vi "Linear Length 1 1721 1853.vi"(6 "Calibration Image":T2, 7 "error in":errorcluster, 8 "ROI 2 Parameters":T9={"ROI 2 Descriptor"={"Global Rectangle"=[], "Contours"=[]}, " ROI 2 Step Size"=10, "ROI 2 Scan Direction"=0, "ROI 2 Process"=enum."Get First + Last Edge", "ROI 2 Edge Options"={"Edge Polarity"=0, "Kernel Size"=3, "Width"=3, "Minimum Edge Strength"=40.0, "Interpolation Type"=enum."Zero Order", "Data Processing Method"=enum."Average"}, "ROI 2 Overlay"=TRUE, "ROI 2 Rake Line Overlay"=TRUE, "ROI 2 Edge/Point Overlay"=TRUE} {"ROI 2 Descriptor"."Contours"."Type" items=["No Selection", "Point", "Line", "Rectangle", "Oval", "Polygon", "Freehand Region", "Annulus", "Unused2", "Unused3", "Broken Line", "Freehand Line", "Rotated Rectangle"]; "ROI 2 Scan Direction" items=["Left To Right", "Right To Left", "Top To Bottom", "Bottom To Top"]; "ROI 2 Edge Options"."Edge Polarity" items=["All Edges", "Rising Edges", "Falling Edges"]; "ROI 2 Edge Options"."Minimum Edge Strength" format="%.2f"; "ROI 2 Edge Options"."Width" step=2; "ROI 2 Edge Options"."Kernel Size" step=2}, 9 "ROI 1 Parameters":T7={"ROI 1 Descriptor"={"Global Rectangle"=[], "Contours"=[]}, "ROI 1 Line Options"={"Number of Lines"=1, "Type"=enum."Best Edge Rake", "Min. Score"=10.0, "Max. Score"=1000.0, "Orientation"=0.0, "Angle Range"=10.0, "Angle Tolerance"=1.0, "Step Size"=5, "Min. SNR (db)"=0.0, "Min. Points (%)"=25.0, "Hough Iterations"=5}, "ROI 1 Edge Options"={"Edge Polarity"=2, "Kernel Size"=3, "Width"=3, "Minimum Edge Strength"=25.0, "Interpolation Type"=enum."Zero Order", "Data Processing Method"=enum."Average"}, "ROI 1 Search Direction"=1, "ROI 1 Overlay"=TRUE, "ROI 1 Rake Line Overlay"=TRUE, "ROI 1 Edge/Point Overlay"=TRUE} {"ROI 1 Descriptor"."Contours"."Type" items=["No Selection", "Point", "Line", "Rectangle", "Oval", "Polygon", "Free", "Annulus", "Unused2", "Unused3", "Broken Line", "Free Hand Line", "Rotated Rectangle"]; "ROI 1 Line Options"."Min. Points (%)" min=0.0 max=100.0; "ROI 1 Line Options"."Min. SNR (db)" min=0.0; "ROI 1 Line Options"."Max. Score" min=0.0 max=1024.0; "ROI 1 Line Options"."Min. Score" min=0.0 max=1024.0 step=1.0; "ROI 1 Edge Options"."Edge Polarity" items=["All Edges", "Rising Edges", "Falling Edges"]; "ROI 1 Edge Options"."Minimum Edge Strength" format="%.2f"; "ROI 1 Edge Options"."Width" step=2; "ROI 1 Edge Options"."Kernel Size" step=2; "ROI 1 Search Direction" items=["Left to Right", "Right to Left", "Top to Bottom", "Bottom to Top"]}, 10 "Input Image":T2) -> (0 "error  out":errorcluster, 1 "Overlay Arrow Lines":T1, 2 "L Outputs":T10, 3 "Refnum out":T2(plugin-control))   [LabVIEW 2019, in "Algorithm.lvclass"]
doc: "Using L advance Line ROI and L advance Search Direction find straight line.\nFind 2 Left Corner Edge points using Rake3 with right inputs. Again find left corner point between these points.\nCalculate perpendicular distance from this point to the line."
uses:
  FrameworkOverrides/Algorithm.lvclass
  <vilib>/vision/NI_Vision_Development_Module.lvlib
  <vilib>/vision/Measure.llb/Edge Polarity.ctl
  <vilib>/vision/Measure.llb/Edge Options.ctl
  <vilib>/vision/Measure.llb/Straight Edge Process.ctl
  <vilib>/vision/Measure.llb/Straight Edge Options.ctl
  <vilib>/vision/Image Controls.llb/IMAQ Image.ctl
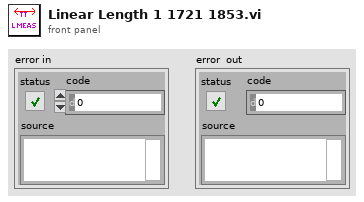
[diagram p1: front panel]
types:
  T1 = cluster{"First Overlay Line ":cluster{"Start Point":cluster{"X":sgl, "Y":sgl}, "Start Point":cluster{"X":sgl, "Y":sgl}}, "Second Overlay Line ":cluster{"Start Point":cluster{"X":sgl, "Y":sgl}, "Start Point":cluster{"X":sgl, "Y":sgl}}}
  T2 = typedef "IMAQ Image.ctl" = refnum<image>
  T3 = typedef "Straight Edge Options.ctl" = cluster{"Number of Lines":i32, "Type":T4, "Min. Score":dbl, "Max. Score":dbl, "Orientation":dbl, "Angle Range":dbl, "Angle Tolerance":dbl, "Step Size":u32, "Min. SNR (db)":dbl, "Min. Points (%)":dbl, "Hough Iterations":i32}
  T4 = typedef "Straight Edge Process.ctl" = enum32{"First Edge Rake", "Best Edge Rake", "Hough Edge Rake", "First Edge Projection", "Best Edge Projection"}
  T5 = typedef "Edge Options.ctl" = cluster{"Edge Polarity":T6, "Kernel Size":u32, "Width":u32, "Minimum Edge Strength":sgl, "Interpolation Type":enum32{"Zero Order", "Bilinear", "Quadratic", "Cubic", "Bilinear Fixed"}, "Data Processing Method":enum32{"Average", "Median"}}
  T6 = typedef "Edge Polarity.ctl" = u32
  T7 = cluster{"ROI 1 Descriptor":cluster{"Global Rectangle":i32[], "Contours":cluster{"ID":enum32{"External", "Internal"}, "Type":u32, "Coordinates":i32[]}[]}, "ROI 1 Line Options":T3, "ROI 1 Edge Options":T5, "ROI 1 Search Direction":u32, "ROI 1 Overlay":bool, "ROI 1 Rake Line Overlay":bool, "ROI 1 Edge/Point Overlay":bool}
  T8 = typedef "ROI Descriptor" = cluster{"Global Rectangle":i32[], "Contours":cluster{"ID":enum32{"External", "Internal"}, "Type":u32, "Coordinates":i32[]}[]}
  T9 = cluster{"ROI 2 Descriptor":T8, " ROI 2 Step Size":u32, "ROI 2 Scan Direction":u16, "ROI 2 Process":enum16{"Get First Edge", "Get First + Last Edge", "Get All Edges", "Get Best Edge"}, "ROI 2 Edge Options":T5, "ROI 2 Overlay":bool, "ROI 2 Rake Line Overlay":bool, "ROI 2 Edge/Point Overlay":bool}
  T10 = cluster{"L":dbl, "Line Coordinates":cluster{"Point1":cluster{"X":sgl, "Y":sgl}, "Point2":cluster{"X":sgl, "Y":sgl}}}
  T11 = enum16{"Get First Edge", "Get First + Last Edge", "Get All Edges", "Get Best Edge"}
  T12 = typedef "IMAQ Rectangle" = cluster{"Left":i32, "Top":i32, "Right":i32, "Bottom":i32, "Rotation":dbl}
  T13 = cluster{"Point 1":cluster{"X":sgl, "Y":sgl}, "Point 2":cluster{"X":sgl, "Y":sgl}}
  T14 = cluster{"Global Rectangle":i32[], "Contours":cluster{"ID":enum32{"External", "Internal"}, "Type":u32, "Coordinates":i32[]}[]}
  T15 = cluster{"Point1 (Pixels)":cluster{"X":sgl, "Y":sgl}, "Point2 (Pixels)":cluster{"X":sgl, "Y":sgl}, "Point1 (Real-World)":cluster{"X":sgl, "Y":sgl}, "Point2 (Real-World)":cluster{"X":sgl, "Y":sgl}, "Angle (Pixel)":dbl, "Angle (Real-World)":dbl, "Score":dbl, "Straightness":dbl, "Average SNR (db)":dbl, "Calibration Valid":bool}[]
  T16 = typedef "Search Line.ctl" = cluster{"Start Point":cluster{"X":sgl, "Y":sgl}, "End Point":cluster{"X":sgl, "Y":sgl}, "Edge Info":T17[], "Edge Map":dbl[], "Calibration Valid":bool}
  T17 = typedef "Edge New.ctl" = cluster{"Location (Pixel)":cluster{"X":sgl, "Y":sgl}, "Location (Real-World)":cluster{"X":sgl, "Y":sgl}, "Distance (Pixel)":dbl, "Distance (Real-World)":dbl, "Strength":dbl, "Noise":dbl, "Rising?":bool}
  T18 = cluster{"Point1 (Pixels)":cluster{"X":sgl, "Y":sgl}, "Point2 (Pixels)":cluster{"X":sgl, "Y":sgl}, "Point1 (Real-World)":cluster{"X":sgl, "Y":sgl}, "Point2 (Real-World)":cluster{"X":sgl, "Y":sgl}, "Angle (Pixel)":dbl, "Angle (Real-World)":dbl, "Score":dbl, "Straightness":dbl, "Average SNR (db)":dbl, "Calibration Valid":bool}
  T19 = cluster{cluster{sgl, "Y":sgl}, "Point 1":cluster{"X":sgl, "Y":sgl}}
  T20 = cluster{"Point 1":cluster{"X":sgl, "Y":sgl}, cluster{sgl, "Y":sgl}}
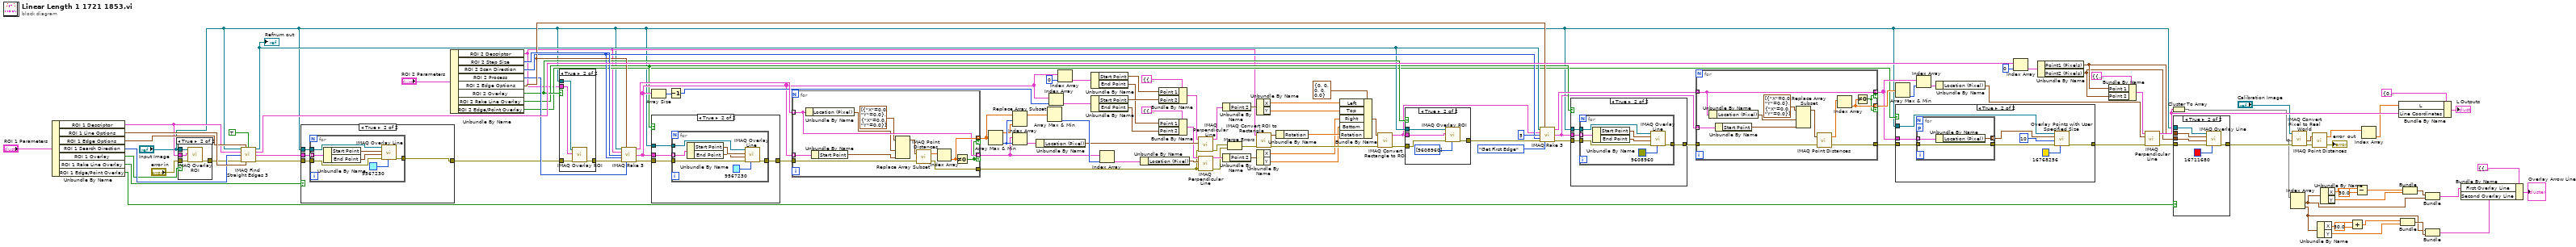
[diagram p0: block diagram]
diagram:
  n1 = Unbundle By Name("ROI 1 Parameters") -> ("ROI 1 Descriptor"=w22:T14, "ROI 1 Line Options"=w64:T3, "ROI 1 Edge Options"=w57:T5, "ROI 1 Search Direction"=w63:u32, "ROI 1 Overlay"=w56:bool, "ROI 1 Rake Line Overlay"=w46:bool, "ROI 1 Edge/Point Overlay"=w30:bool)
  n2 = case shown="True" w56 {
    tunnel: "error in" -> [w122 w126]
    tunnel: [w122 w125] -> w58
    tunnel: "Input Image" -> [_ w124]
    tunnel: w22 -> [_ w123]
    frame False {
    }
    frame True {
      n3 = call "IMAQ Overlay ROI"("error in (no error)"=w126, "ROI Descriptor"=w123, "Image"=w124) -> ("error out"=w125:errorcluster)  [unwired: 7 in, 1 out]
    }
  }
  n4 = call "IMAQ Find Straight Edges 3"("Image"="Input Image", "Edge Options"=w57, "Optimized Mode"=TRUE, "ROI Descriptor"=w22, "Search Direction"=w63, "error in (no error)"=w58, "Line Options"=w64) -> ("Image (duplicate)"=w53:T2, "Straight Edges"=w121:T15, "Search Lines Information"=w49:T16[], "error out"=w48:errorcluster)  [unwired: 4 in, 1 out]
  "Refnum out" <- w53
  n5 = case shown="True" w46 {
    tunnel: w49 -> [_ w131]
    tunnel: "Input Image" -> [_ w130]
    tunnel: w48 -> [w127 w129]
    tunnel: [w127 w128] -> w47
    frame False {
    }
    frame True {
      n6 = for {
        tunnel: w131 -> [w138] mode=indexing
        tunnel: w130 -> [w135]
        tunnel: w129 -> [w134]
        tunnel: [w133] -> w128
        n7 = Unbundle By Name(w138) -> ("Start Point"=w137:cluster{"X":sgl, "Y":sgl}, "End Point"=w136:cluster{"X":sgl, "Y":sgl})
        n8 = call "IMAQ Overlay Line"("Color"=u32 9567230, "error in (no error)"=w134, "End Point"=w136, "Start Point"=w137, "Image"=w135) -> ("error out"=w133:errorcluster)  [unwired: 5 in, 1 out]
      }
    }
  }
  n9 = Unbundle By Name("ROI 2 Parameters") -> ("ROI 2 Descriptor"=w21:T8, "ROI 2 Step Size"=w62:u32, "ROI 2 Scan Direction"=w60:u16, "ROI 2 Process"=w59:T11, "ROI 2 Edge Options"=w61:T5, "ROI 2 Overlay"=w54:bool, "ROI 2 Rake Line Overlay"=w42:bool, "ROI 2 Edge/Point Overlay"=w37:bool)
  n10 = case shown="True" w54 {
    tunnel: w47 -> [w139 w143]
    tunnel: [w139 w142] -> w55
    tunnel: "Input Image" -> [_ w141]
    tunnel: w21 -> [_ w140]
    frame False {
    }
    frame True {
      n11 = call "IMAQ Overlay ROI"("error in (no error)"=w143, "ROI Descriptor"=w140, "Image"=w141) -> ("error out"=w142:errorcluster)  [unwired: 7 in, 1 out]
    }
  }
  n12 = call "IMAQ Rake 3"("Image"="Input Image", "Edge Options"=w61, "ROI Descriptor"=w21, "Step Size"=w62, "Scan Direction"=w60, "error in (no error)"=w55, "Process"=w59) -> ("First Edges"=w120:T17[], "Search Lines"=w45:T16[], "error out"=w44:errorcluster)  [unwired: 5 in, 1 out]
  n13 = Array Size(array=w45) -> (size(s)=w97:i32)
  n14 = case shown="True" w42 {
    tunnel: w45 -> [_ w148]
    tunnel: "Input Image" -> [_ w147]
    tunnel: w44 -> [w144 w146]
    tunnel: [w144 w145] -> w43
    frame False {
    }
    frame True {
      n15 = for {
        tunnel: w148 -> [w155] mode=indexing
        tunnel: w147 -> [w152]
        tunnel: w146 -> [w151]
        tunnel: [w150] -> w145
        n16 = Unbundle By Name(w155) -> ("Start Point"=w154:cluster{"X":sgl, "Y":sgl}, "End Point"=w153:cluster{"X":sgl, "Y":sgl})
        n17 = call "IMAQ Overlay Line"("Color"=u32 9567230, "error in (no error)"=w151, "End Point"=w153, "Start Point"=w154, "Image"=w152) -> ("error out"=w150:errorcluster)  [unwired: 5 in, 1 out]
      }
    }
  }
  n18 = Decrement(x=w97) -> (x-1=w96:i32)
  n19 = for {
    tunnel: w45 -> [w166] mode=indexing
    tunnel: w120 -> [w161] mode=indexing
    tunnel: [w162] -> w106 mode=indexing if=w160
    tunnel: w43 -> [w164]
    tunnel: [w163] -> w70
    tunnel: [w161] -> w101 mode=indexing if=w160
    n20 = Unbundle By Name(w161) -> ("Location (Pixel)"=w158:cluster{"X":sgl, "Y":sgl})
    n21 = Unbundle By Name(w166) -> ("Start Point"=w157:cluster{"X":sgl, "Y":sgl})
    n22 = Replace Array Subset(array=cluster{"X":sgl, "Y":sgl}[] [{"X"=0.0, "Y"=0.0}, {"X"=0.0, "Y"=0.0}] ("appended array"), new element #1=w158, new element #2=w157) -> (w156:cluster{"X":sgl, "Y":sgl}[])  [unwired: 2 in]
    n23 = call "IMAQ Point Distances"("Points"=w156, "error in (no error)"=w164) -> ("Distances"=w165:sgl[], "error out"=w163:errorcluster)  [unwired: 3 in]
    n24 = Index Array(array=w165) -> (element=w162:sgl)  [unwired: 1 in]
    n25 = Not Equal To 0?(x=w162) -> (x != 0?=w160:bool)
  }
  n26 = Array Max & Min(array=w106) -> (max value=w104:sgl, min index (indices)=w105:i32)  [unwired: 2 out]
  n27 = Replace Array Subset(array=w106, new element=w104, index=w105) -> (w103:sgl[])
  n28 = Index Array(array=w101, index=w105) -> (element=w119:T17)
  n29 = Unbundle By Name(w119) -> ("Location (Pixel)"=w94:cluster{"X":sgl, "Y":sgl})
  n30 = Array Max & Min(array=w103) -> (min index (indices)=w102:i32)  [unwired: 3 out]
  n31 = Index Array(array=w45, index=w96) -> (element=w95:T16)
  n32 = Index Array(array=w45, index=0) -> (element=w99:T16)
  n33 = Unbundle By Name(w99) -> ("Start Point"=w92:cluster{"X":sgl, "Y":sgl}, "End Point"=w88:cluster{"X":sgl, "Y":sgl})
  n34 = Unbundle By Name(w95) -> ("Start Point"=w91:cluster{"X":sgl, "Y":sgl}, "End Point"=w87:cluster{"X":sgl, "Y":sgl})
  n35 = Index Array(array=w101, index=w102) -> (element=w98:T17)
  n36 = Unbundle By Name(w98) -> ("Location (Pixel)"=w85:cluster{"X":sgl, "Y":sgl})
  n37 = Bundle By Name(cluster=T13 {"Point 1"={"X"=0.0, "Y"=0.0}, "Point 2"={"X"=0.0, "Y"=0.0}} ("Line"), "Point 1"=w92, "Point 2"=w91) -> (w90:T13)
  n38 = Bundle By Name(cluster=T13 {"Point 1"={"X"=0.0, "Y"=0.0}, "Point 2"={"X"=0.0, "Y"=0.0}} ("Line"), "Point 1"=w88, "Point 2"=w87) -> (w86:T13)
  n39 = call "IMAQ Perpendicular Line"("error in (no error)"=w70, "Point"=w94, "Line"=w90) -> ("error out"=w78:errorcluster, "Perpendicular Line"=w89:T13)  [unwired: 6 in, 1 out]
  n40 = call "IMAQ Perpendicular Line"("error in (no error)"=w70, "Point"=w85, "Line"=w86) -> ("error out"=w77:errorcluster, "Perpendicular Line"=w83:T13)  [unwired: 6 in, 1 out]
  n41 = Unbundle By Name(w89) -> ("Point 2"=w26:cluster{"X":sgl, "Y":sgl})
  n42 = Unbundle By Name(w83) -> ("Point 2"=w29:cluster{"X":sgl, "Y":sgl})
  n43 = Merge Errors(w78, w77) -> (w76:errorcluster)
  n44 = Unbundle By Name(w26) -> ("X"=w25:sgl, "Y"=w24:sgl)
  n45 = call "IMAQ Convert ROI to Rectangle"("error in (no error)"=w76, "ROI Descriptor"=w21) -> ("error out"=w81:errorcluster, "Rectangle"=w80:T12)  [unwired: 7 in]
  n46 = Unbundle By Name(w29) -> ("X"=w28:sgl, "Y"=w27:sgl)
  n47 = Unbundle By Name(w80) -> ("Rotation"=w79:dbl)
  n48 = Bundle By Name(cluster=T12 {"Left"=0, "Top"=0, "Right"=0, "Bottom"=0, "Rotation"=0.0} ("Rectangle"), "Left"=w25, "Top"=w24, "Right"=w28, "Bottom"=w27, "Rotation"=w79) -> (w75:T12)
  n49 = call "IMAQ Convert Rectangle to ROI"("error in (no error)"=w81, "Rectangle"=w75) -> ("error out"=w51:errorcluster, "ROI Descriptor"=w52:T8)  [unwired: 7 in]
  n50 = case shown="True" w54 {
    tunnel: w51 -> [w167 w172]
    tunnel: [w167 w171] -> w50
    tunnel: w53 -> [_ w170]
    tunnel: w52 -> [_ w169]
    frame False {
    }
    frame True {
      n51 = call "IMAQ Overlay ROI"("Colors (Green)"=u32[] [9608960], "error in (no error)"=w172, "ROI Descriptor"=w169, "Image"=w170) -> ("error out"=w171:errorcluster)  [unwired: 6 in, 1 out]
    }
  }
  n52 = call "IMAQ Rake 3"("Image"=w53, "Edge Options"=w61, "ROI Descriptor"=w52, "Step Size"=u32 5, "Scan Direction"=w60, "error in (no error)"=w50, "Process"=T11."Get First Edge") -> ("First Edges"=w74:T17[], "Search Lines"=w41:T16[], "error out"=w40:errorcluster)  [unwired: 5 in, 1 out]
  n53 = case shown="True" w42 {
    tunnel: w41 -> [_ w177]
    tunnel: "Input Image" -> [_ w176]
    tunnel: w40 -> [w173 w175]
    tunnel: [w173 w174] -> w39
    frame False {
    }
    frame True {
      n54 = for {
        tunnel: w177 -> [w184] mode=indexing
        tunnel: w176 -> [w181]
        tunnel: w175 -> [w180]
        tunnel: [w179] -> w174
        n55 = Unbundle By Name(w184) -> ("Start Point"=w183:cluster{"X":sgl, "Y":sgl}, "End Point"=w182:cluster{"X":sgl, "Y":sgl})
        n56 = call "IMAQ Overlay Line"("Color"=u32 9608960, "error in (no error)"=w180, "End Point"=w182, "Start Point"=w183, "Image"=w181) -> ("error out"=w179:errorcluster)  [unwired: 5 in, 1 out]
      }
    }
  }
  n57 = for {
    tunnel: w41 -> [w195] mode=indexing
    tunnel: w74 -> [w190] mode=indexing
    tunnel: [w191] -> w72 mode=indexing if=w189
    tunnel: w39 -> [w193]
    tunnel: [w192] -> w36
    tunnel: [w190] -> w38 mode=indexing if=w189
    n58 = Unbundle By Name(w190) -> ("Location (Pixel)"=w187:cluster{"X":sgl, "Y":sgl})
    n59 = Unbundle By Name(w195) -> ("Start Point"=w186:cluster{"X":sgl, "Y":sgl})
    n60 = Replace Array Subset(array=cluster{"X":sgl, "Y":sgl}[] [{"X"=0.0, "Y"=0.0}, {"X"=0.0, "Y"=0.0}] ("appended array"), new element #1=w187, new element #2=w186) -> (w185:cluster{"X":sgl, "Y":sgl}[])  [unwired: 2 in]
    n61 = call "IMAQ Point Distances"("Points"=w185, "error in (no error)"=w193) -> ("Distances"=w194:sgl[], "error out"=w192:errorcluster)  [unwired: 3 in]
    n62 = Index Array(array=w194) -> (element=w191:sgl)  [unwired: 1 in]
    n63 = Not Equal To 0?(x=w191) -> (x != 0?=w189:bool)
  }
  n64 = Array Max & Min(array=w72) -> (min index (indices)=w71:i32)  [unwired: 3 out]
  n65 = case shown="True" w37 {
    tunnel: w38 -> [_ w204]
    tunnel: "Input Image" -> [_ w202]
    tunnel: w36 -> [w196 w199]
    tunnel: [w196 w197] -> w35
    frame False {
    }
    frame True {
      n66 = for {
        tunnel: w204 -> [w207] mode=indexing
        tunnel: [w206] -> w203 mode=indexing
        workers-P: _ -> [_]
        tunnel: w199 -> [w205]
        tunnel: [w205] -> w198
        n67 = Unbundle By Name(w207) -> ("Location (Pixel)"=w206:cluster{"X":sgl, "Y":sgl})
      }
      n68 = call "Overlay Points with User Specified Size.vi"("Color"=u32 16768256, "error in"=w198, "Point Diameter (5)"=u32 10, "Points"=w203, "Image In"=w202) -> ("error out"=w197:errorcluster)  [unwired: 5 in, 1 out]
    }
  }
  n69 = Index Array(array=w38, index=w71) -> (element=w73:T17)
  n70 = Unbundle By Name(w73) -> ("Location (Pixel)"=w69:cluster{"X":sgl, "Y":sgl})
  n71 = Index Array(array=w121, index=0) -> (element=w114:T18)
  n72 = Unbundle By Name(w114) -> ("Point1 (Pixels)"=w34:cluster{"X":sgl, "Y":sgl}, "Point2 (Pixels)"=w33:cluster{"X":sgl, "Y":sgl})
  n73 = Bundle By Name(cluster=T13 {"Point 1"={"X"=0.0, "Y"=0.0}, "Point 2"={"X"=0.0, "Y"=0.0}} ("Line"), "Point 1"=w34, "Point 2"=w33) -> (w112:T13)
  n74 = call "IMAQ Perpendicular Line"("error in (no error)"=w35, "Point"=w69, "Line"=w112) -> ("error out"=w32:errorcluster, "Perpendicular Line"=w111:T13)  [unwired: 6 in, 1 out]
  n75 = Cluster To Array(cluster=w111) -> (array=w17:cluster{"X":sgl, "Y":sgl}[])
  n76 = case shown="True" w30 {
    tunnel: w34 -> [_ w214]
    tunnel: w33 -> [_ w213]
    tunnel: "Input Image" -> [_ w211]
    tunnel: w32 -> [w208 w210]
    tunnel: [w208 w209] -> w31
    frame False {
    }
    frame True {
      n77 = call "IMAQ Overlay Line"("Color"=u32 16711680, "error in (no error)"=w210, "End Point"=w213, "Start Point"=w214, "Image"=w211) -> ("error out"=w209:errorcluster)  [unwired: 5 in, 1 out]
    }
  }
  n78 = Index Array(array=w17) -> (element #1=w11:cluster{"X":sgl, "Y":sgl}, element #2=w2:cluster{"X":sgl, "Y":sgl})  [unwired: 2 in]
  n79 = call "IMAQ Convert Pixel to Real World"("error in (no error)"=w31, "Array of Pixel Coordinates"=w17, "Calibrated Image"="Calibration Image") -> ("error out"=w108:errorcluster, "Array of Real World Coordinates"=w110:cluster{"X":sgl, "Y":sgl}[])  [unwired: 3 in, 4 out]
  n80 = call "IMAQ Point Distances"("Points"=w110, "error in (no error)"=w108) -> ("Distances"=w109:sgl[], "error out"=→"error  out":errorcluster)  [unwired: 3 in]
  n81 = Unbundle By Name(w2) -> ("X"=w7:sgl, "Y"=w5:sgl)
  n82 = Unbundle By Name(w11) -> ("X"=w16:sgl, "Y"=w12:sgl)
  n83 = Add(x=w7, y=sgl 30.0) -> (x+y=w4:sgl)
  n84 = Subtract(x=w16, y=sgl 30.0) -> (x-y=w14:sgl)
  n85 = Index Array(array=w109) -> (element=w107:sgl)  [unwired: 1 in]
  n86 = Bundle By Name(cluster=T10 {"L"=0.0, "Line Coordinates"={"Point1"={"X"=0.0, "Y"=0.0}, "Point2"={"X"=0.0, "Y"=0.0}}}, "L"=w107, "Line Coordinates"=w111) -> (→"L Outputs":T10)
  n87 = Bundle(w4, "Y"=w5) -> (w3:cluster{sgl, "Y":sgl})  [unwired: 1 in]
  n88 = Bundle(w14, "Y"=w12) -> (w10:cluster{sgl, "Y":sgl})  [unwired: 1 in]
  n89 = Bundle(w10, "Point 1"=w11) -> (w9:T19)  [unwired: 1 in]
  n90 = Bundle("Point 1"=w2, w3) -> (w1:T20)  [unwired: 1 in]
  n91 = Bundle By Name(cluster=T1 {"First Overlay Line "={"Start Point"={"X"=0.0, "Y"=0.0}, "Start Point"={"X"=0.0, "Y"=0.0}}, "Second Overlay Line "={"Start Point"={"X"=0.0, "Y"=0.0}, "Start Point"={"X"=0.0, "Y"=0.0}}} ("Overlay Arrow Lines"), "First Overlay Line"=w9, "Second Overlay Line"=w1) -> (→"Overlay Arrow Lines":T1)
